vi "Get Time Data.vi"(0 "reference in":refnum<class "WaveFile.lvclass">, 5 "error in (no error)":errorcluster) -> (11 "Time data ref":refnum<class "GSwFormDSP.lvclass">, 13 "wForms":waveform(dbl)[](array[waveform]), 14 "reference out":refnum<class "WaveFile.lvclass">, 19 "error out":errorcluster)   [LabVIEW 2022 SP3, in "WaveFile.lvclass"]
uses:
  WaveFile.lvclass
  API/GSwFormDSP_class/GSwFormDSP.lvclass
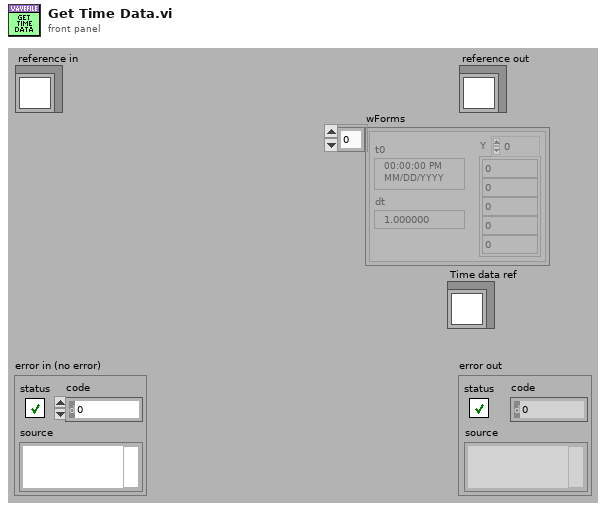
[diagram p1: front panel]
types:
  T1 = typedef "WaveFile.lvclass/ObjectAttributes.ctl" = cluster{"Time Data":refnum<class "GSwFormDSP.lvclass">, "New Time Data Obj?":bool, "NIST File Header":T2}
  T2 = typedef "WaveFile.lvclass/NIST File Header.ctl" = cluster{"Version":string, "Header Nb Bytes":i32, "Nb Samples":i32, "Nb Bytes/sample":i32, "Nb Channels":i32, "byte order":enum16{"big-endian, network order", "native, host order", "little-endian"}, "Fs":dbl, "Valid Header?":bool}
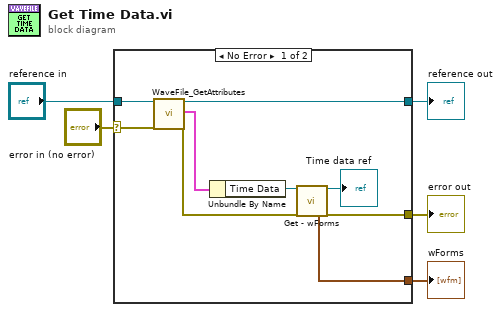
[diagram p0: block diagram]
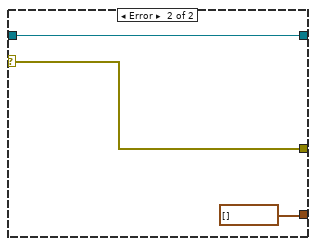
[diagram p2: hidden frame]
diagram:
  n1 = case shown="No Error" "error in (no error)" {
    selector: "error in (no error)" -> [w14 w17]
    tunnel: [w7 w17] -> w4
    tunnel: [w13 w16] -> w2
    tunnel: "reference in" -> [w11 w16]
    tunnel: [w6 waveform(dbl)[] [] ("wForms")] -> w1
    frame No Error {
      n2 = call "WaveFile_GetAttributes.vi"("reference in"=w11, "error in (no error)"=w14) -> ("reference out"=w13:refnum<class "WaveFile.lvclass">, "attributes"=w12:T1, "error out"=w8:errorcluster)  [unwired: 14 in, 1 out]
      n3 = Unbundle By Name(w12) -> ("Time Data"=w10:refnum<class "GSwFormDSP.lvclass">)
      n4 = call-dynamic "Get - wForms.vi"("reference in"=w10, "error in (no error)"=w8) -> ("wForms"=w6:waveform(dbl)[], "reference out"=→"Time data ref":refnum<class "GSwFormDSP.lvclass">, "error out"=w7:errorcluster)  [unwired: 14 in, 1 out]
    }
    frame Error {
    }
  }
  "error out" <- w4
  "reference out" <- w2
  "wForms" <- w1
